vi "formula.vi"(10 "Conversion\nToggle":bool, 11 "Input Temperature\nin Celsius in":dbl) -> (3 "Input Temperature\nin Celsius out":dbl)   [LabVIEW 2023]
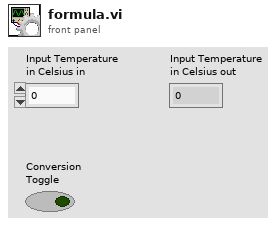
[diagram p1: front panel]
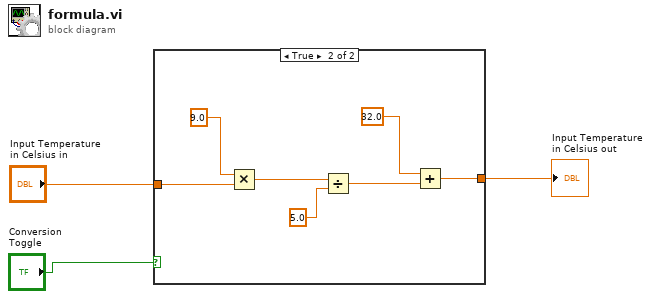
[diagram p0: block diagram]
diagram:
  n1 = case shown="True" "Conversion\nToggle" {
    tunnel: "Input Temperature\nin Celsius in" -> [w4 w11]
    tunnel: [w4 w5] -> w2
    frame False {
    }
    frame True {
      n2 = Multiply(x=9.0, y=w11) -> (x*y=w7:dbl)
      n3 = Divide(x=w7, y=5.0) -> (x/y=w9:dbl)
      n4 = Add(x=32.0, y=w9) -> (x+y=w5:dbl)
    }
  }
  "Input Temperature\nin Celsius out" <- w2
